vi "initialise.vi"(8 "error in (no error)":errorcluster, 10 "main_app_instance":bool, 11 "WinX32Camera in":refnum<class "WinX32Camera.lvclass">) -> (0 "error out":errorcluster, 3 "WinX32Camera out":refnum<class "WinX32Camera.lvclass">)   [LabVIEW 2011, in "WinX32Camera.lvclass"]
uses:
  WinX32Camera.lvclass
  WinX32Camera.lvclass/WinX32Camera.ctl
panel:
  in  "WINX32Lib.IDocFile":refnum<k7>
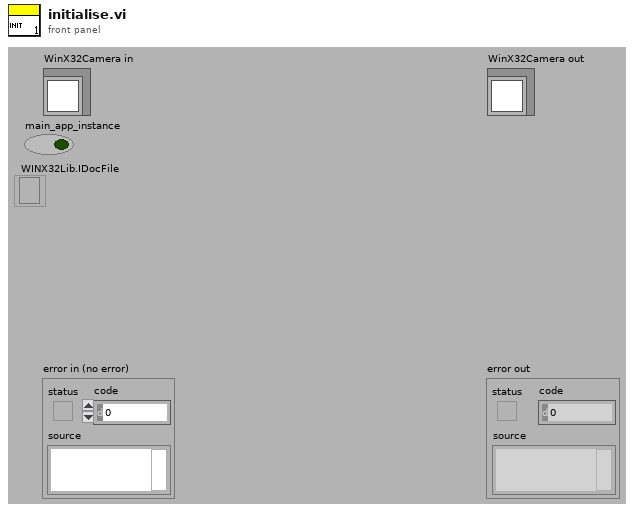
[diagram p1: front panel]
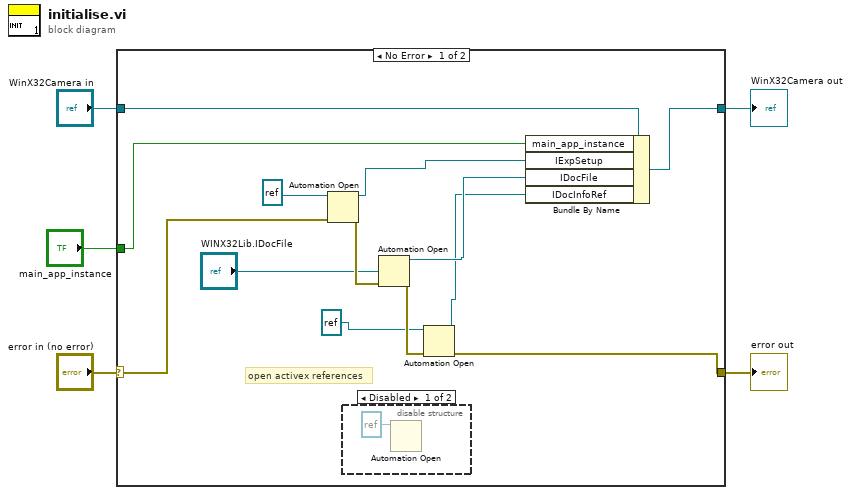
[diagram p0: block diagram]
diagram:
  n1 = case shown="No Error" "error in (no error)" {
    selector: "error in (no error)" -> [w15 w21]
    tunnel: [w11 w21] -> w4
    tunnel: [w16 w20] -> w2
    tunnel: "WinX32Camera in" -> [w17 w20]
    tunnel: "main_app_instance" -> [w18 _]
    frame No Error {
      # "open activex references"
      n2 = Automation Open(error in (no error)=w15, Automation Refnum=refnum<k7> refnum ("IExpSetup")) -> (Automation Refnum=w9:refnum<k7>, error out=w14:errorcluster)  [unwired: 2 in]
      n3 = disable-structure shown="Disabled" {
        frame Disabled {
          n4 = Automation Open(Automation Refnum=refnum<k7> refnum) -> ()  [unwired: 3 in, 2 out]
        }
        frame Enabled {
        }
      }
      n5 = Automation Open(error in (no error)=w14, Automation Refnum="WINX32Lib.IDocFile") -> (Automation Refnum=w13:refnum<k7>, error out=w12:errorcluster)  [unwired: 2 in]
      n6 = Automation Open(error in (no error)=w12, Automation Refnum=refnum<k7> refnum ("IDocInfoRef")) -> (Automation Refnum=w7:refnum<k7>, error out=w11:errorcluster)  [unwired: 2 in]
      n7 = Bundle By Name(cluster=w17, "main_app_instance"=w18, "IExpSetup"=w9, "IDocFile"=w13, "IDocInfoRef"=w7) -> (w16:refnum<class "WinX32Camera.lvclass">)
    }
    frame Error {
    }
  }
  "error out" <- w4
  "WinX32Camera out" <- w2
